vi "Workspace.Path.RemoveIP.vi"(11 "CD Path":string) -> (1 "Name":string, 3 "Path":string)   [LabVIEW 2019, in "Diagnostics Workspace Shared.lvlib"]
uses:
  NationalInstruments.VeriStand
  Diagnostics Workspace Shared.lvlib
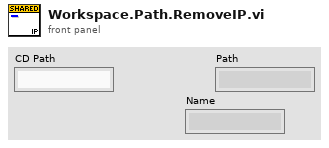
[diagram p1: front panel]
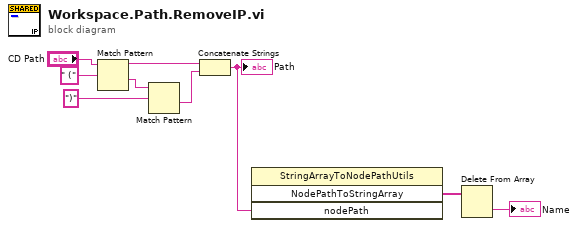
[diagram p0: block diagram]
diagram:
  n1 = Match Pattern(string="CD Path", regular expression=" (") -> (before substring=w8:string, after substring=w6:string)  [unwired: 1 in, 2 out]
  n2 = Match Pattern(string=w6, regular expression=")") -> (after substring=w7:string)  [unwired: 1 in, 3 out]
  n3 = Concatenate Strings(w8, w7) -> (w3:string)
  "Path" <- w3
  n4 = invoke class="StringArrayToNodePathUtils" method="NodePathToStringArray"("nodePath"=w3) -> ("NodePathToStringArray"=w2:string[])  [unwired: 3 in, 3 out]
  n5 = Delete From Array(array=w2) -> (deleted portion=→"Name":string)  [unwired: 2 in, 1 out]
